vi "Configure OCP.vi"(8 "error in (no error)":errorcluster, 9 "Over Current Protection (0.0 V)":dbl format="%.2g", 11 "VISA resource name":refnum<visa-resource-name>) -> (0 "error out":errorcluster, 3 "VISA resource name out":refnum<visa-resource-name>)   [LabVIEW 2022 SP3, in "BK Precision 9103.lvlib"]
doc: "Configures over current protection (OCP) of the power supply."
uses:
  <instrlib>/BK Precision 9103/BK Precision 9103.lvlib
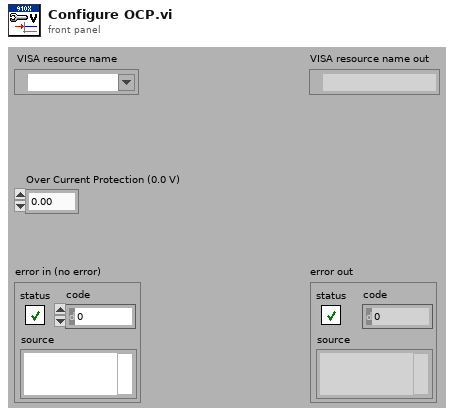
[diagram p1: front panel]
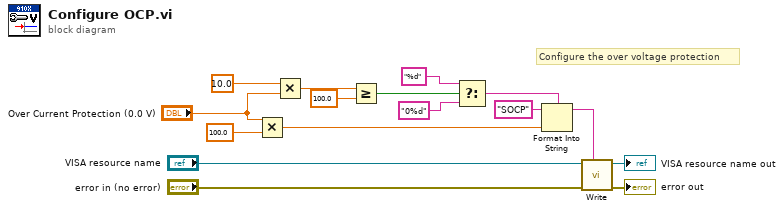
[diagram p0: block diagram]
diagram:
  # "Configure the over voltage protection"
  n1 = Multiply(x="Over Current Protection (0.0 V)", y=100.0) -> (x*y=w9:dbl)
  n2 = Multiply(x=10.0 ("y"), y="Over Current Protection (0.0 V)") -> (x*y=w15:dbl)
  n3 = Greater Or Equal?(x=w15, y=100.0) -> (x >= y?=w13:bool)
  n4 = Select(t="%d" ("format string"), s=w13, f="0%d" ("format string")) -> (s? t:f=w6:string)
  n5 = Format Into String(format string=w6, initial string="SOCP", w9) -> (resulting string=w1:string)  [unwired: 1 in, 1 out]
  n6 = call <instrlib>:"Write.vi"("Input String"=w1, "error in (no error)"="error in (no error)", "VISA resource name"="VISA resource name") -> ("error out"=→"error out":errorcluster, "VISA resource name out"=→"VISA resource name out":refnum<visa-resource-name>)  [unwired: 6 in, 1 out]
